vi "To Serial Form.vi"(6 "Serial Version":T1, 10 "Serializer in":refnum<class "Serializer.lvclass">=refnum, 11 "Nicholas Data in":refnum<class "Nicholas Data.lvclass">) -> (0 "error out":errorcluster, 2 "Serializer out":refnum<class "Serializer.lvclass">, 3 "Nicholas Data out":refnum<class "Nicholas Data.lvclass">)   [LabVIEW 2015, in "Nicholas Data.lvclass"]
uses:
  Nicholas Data.lvclass
  <vilib>/NI/AQ Character Lineator/Serializable/Insert Serializable.vi
  Reusable/CRDS/Data/Main/CRDS Data.lvclass
  Reusable/PAS/Data/Main/PAS Data.lvclass
  Devices/TE Cooler/Data/TECData.lvclass
  Devices/Alicat/Session Based/Data/Alicat Data.lvclass
  Reusable/Data/Array Data/Single 1-D/Single_Array.lvclass
  <vilib>/NI/AQ Character Lineator/Serializable/Insert Boolean Array.vi
  Reusable/Data/Data.lvclass
  <vilib>/NI/AQ Character Lineator/Serializer/Serializer.lvclass
  <vilib>/NI/AQ Character Lineator/Serialization Common/Serial Version.ctl
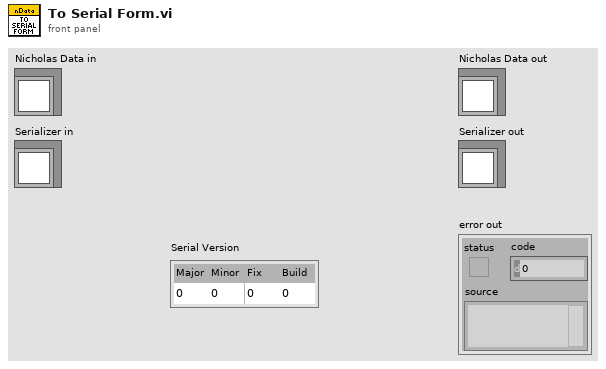
[diagram p1: front panel]
types:
  T1 = typedef "Serialization Common.lvlib/Serial Version.ctl" = cluster{"Major":u16, "Minor":u16, "Fix":u16, "Build":u16}
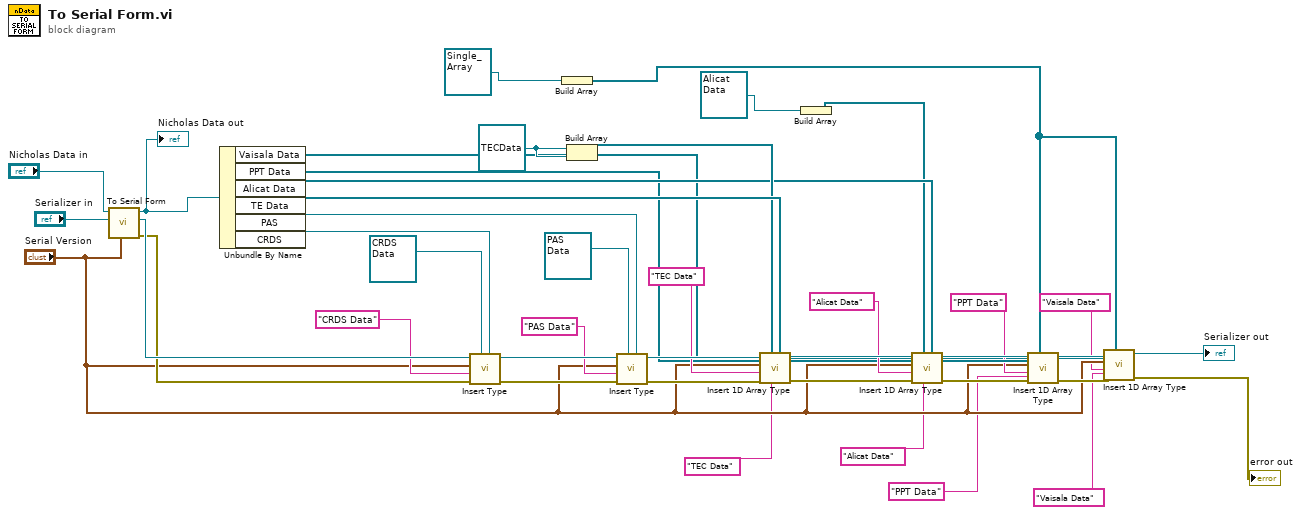
[diagram p0: block diagram]
diagram:
  w25 = refnum<class "TECData.lvclass"> refnum ("TE Cooler.lvlib:TEC Data")
  n1 = call-parent "To Serial Form.vi"("Serial Version"="Serial Version", "Serializer in"="Serializer in", "Data in"="Nicholas Data in") -> ("error out"=w35:errorcluster, "Serializer out"=w40:refnum<class "Serializer.lvclass">, "Data out"=w39:refnum<class "Nicholas Data.lvclass">)  [unwired: 6 in]
  "Nicholas Data out" <- w39
  n2 = Unbundle By Name(w39) -> ("Vaisala Data"=w10:refnum<class "Single_Array.lvclass">[], "PPT Data"=w15:refnum<class "Single_Array.lvclass">[], "Alicat Data"=w22:refnum<class "Alicat Data.lvclass">[], "TE Data"=w28:refnum<class "TECData.lvclass">[], "PAS"=w32:refnum<class "PAS Data.lvclass">, "CRDS"=w38:refnum<class "CRDS Data.lvclass">)
  n3 = call-poly <vilib>:"Insert Type.vi"("Serializable"=w38, "Default Value"=refnum<class "CRDS Data.lvclass"> refnum ("CRDS"), "error in (no error)"=w35, "Name"="CRDS Data", "Serial Version"="Serial Version", "Serializer in"=w40) -> ("error out"=w33:errorcluster, "Serializer out"=w34:refnum<class "Serializer.lvclass">)  [unwired: 4 in]
  n4 = Build Array(refnum<class "Single_Array.lvclass"> refnum ("Base Data Lib:[SGL]")) -> (w9:refnum<class "Single_Array.lvclass">[])
  n5 = Build Array(w25, w25) -> (w24:refnum<class "TECData.lvclass">[])
  n6 = call-poly <vilib>:"Insert Type.vi"("Serializable"=w32, "Default Value"=refnum<class "PAS Data.lvclass"> refnum ("PAS"), "error in (no error)"=w33, "Name"="PAS Data", "Serial Version"="Serial Version", "Serializer in"=w34) -> ("error out"=w26:errorcluster, "Serializer out"=w29:refnum<class "Serializer.lvclass">)  [unwired: 4 in]
  n7 = call-poly <vilib>:"Insert 1D Array Type.vi"("Booleans"=w28, 6:"TEC Data" ("Default Class Qualified Name"), "Default Value"=w24, "error in (no error)"=w26, "Name"="TEC Data", 10:"Serial Version", "Serializer in"=w29) -> ("error out"=w19:errorcluster, "Serializer out"=w23:refnum<class "Serializer.lvclass">)  [unwired: 3 in]
  n8 = Build Array(refnum<class "Alicat Data.lvclass"> refnum ("Alicat Data")) -> (w20:refnum<class "Alicat Data.lvclass">[])
  n9 = call-poly <vilib>:"Insert 1D Array Type.vi"("Booleans"=w22, 6:"Alicat Data" ("Default Class Qualified Name"), "Default Value"=w20, "error in (no error)"=w19, "Name"="Alicat Data", 10:"Serial Version", "Serializer in"=w23) -> ("error out"=w16:errorcluster, "Serializer out"=w17:refnum<class "Serializer.lvclass">)  [unwired: 3 in]
  n10 = call-poly <vilib>:"Insert 1D Array Type.vi"("Booleans"=w15, 6:"PPT Data" ("Default Class Qualified Name"), "Default Value"=w9, "error in (no error)"=w16, "Name"="PPT Data", 10:"Serial Version", "Serializer in"=w17) -> ("error out"=w11:errorcluster, "Serializer out"=w12:refnum<class "Serializer.lvclass">)  [unwired: 3 in]
  n11 = call-poly <vilib>:"Insert 1D Array Type.vi"("Booleans"=w10, 6:"Vaisala Data" ("Default Class Qualified Name"), "Default Value"=w9, "error in (no error)"=w11, "Name"="Vaisala Data", 10:"Serial Version", "Serializer in"=w12) -> ("error out"=→"error out":errorcluster, "Serializer out"=→"Serializer out":refnum<class "Serializer.lvclass">)  [unwired: 3 in]
